vi "Engine In - Sensor - MAT.vi"(10 "Loop Freq [Hz]":sgl, 11 "Raw Intake Manifold Temp [Ohm]":sgl) -> (3 "Intake Manifold Temp [C]":sgl)   [LabVIEW 2015, in "ECS-RT.lvlib"]
uses:
  ECS-RT.lvlib
  <vilib>/ptbypt/NI_PtbyPt.lvlib
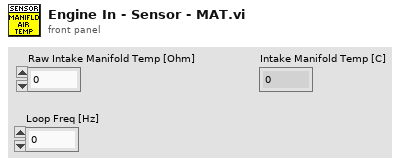
[diagram p1: front panel]
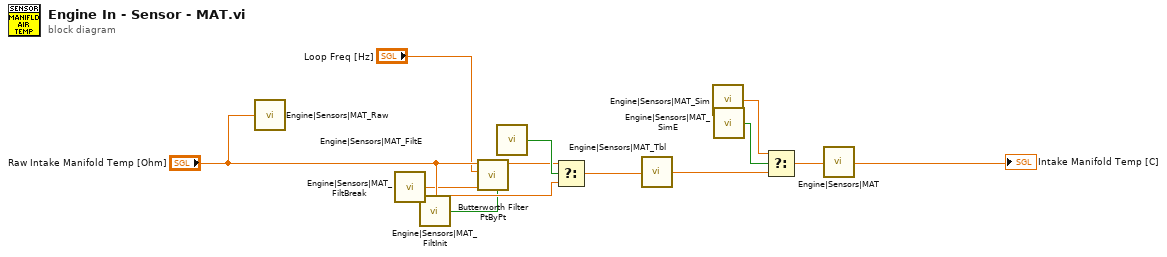
[diagram p0: block diagram]
diagram:
  n1 = call "Engine|Sensors|MAT_Raw"("Value"="Raw Intake Manifold Temp [Ohm]") -> ()
  n2 = call "Engine|Sensors|MAT_FiltBreak"() -> ("Value"=w7:sgl)
  n3 = call "Engine|Sensors|MAT_FiltInit"() -> ("Value"=w5:bool)
  n4 = call <vilib>:"Butterworth Filter PtByPt.vi"("initialize"=w5, "low cutoff freq: fl"=w7, "sampling freq: fs"="Loop Freq [Hz]", "x"="Raw Intake Manifold Temp [Ohm]") -> ("Filtered x"=w6:dbl)  [unwired: 5 in, 1 out]
  n5 = call "Engine|Sensors|MAT_FiltE"() -> ("Value"=w8:bool)
  n6 = Select(t=w6, s=w8, f="Raw Intake Manifold Temp [Ohm]") -> (s? t:f=w3:dbl)
  n7 = call "Engine|Sensors|MAT_Tbl"("X Index"=w3) -> ("Y"=w2:sgl)
  n8 = call "Engine|Sensors|MAT_Sim"() -> ("Value"=w4:sgl)
  n9 = call "Engine|Sensors|MAT_SimE"() -> ("Value"=w9:bool)
  n10 = Select(t=w4, s=w9, f=w2) -> (s? t:f=w11:sgl)
  "Intake Manifold Temp [C]" <- w11
  n11 = call "Engine|Sensors|MAT"("Value"=w11) -> ()
